vi "Read Motor Temperature.vi"(11 "Thermocouple in":refnum<class "Thermocouple.lvclass">) -> (2 "Motor Temperature":dbl[unit]=273.15 min=-614.85 max=1161.15 format="%.6f", 3 "Thermocouple out":refnum<class "Thermocouple.lvclass">)   [LabVIEW 2013, in "Thermocouple.lvclass"]
uses:
  Thermocouple.lvclass
  Thermocouple.lvclass/Thermocouple.ctl
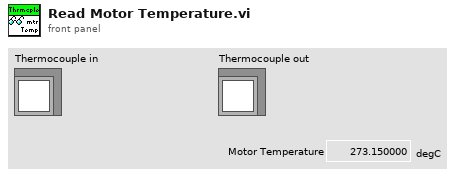
[diagram p1: front panel]
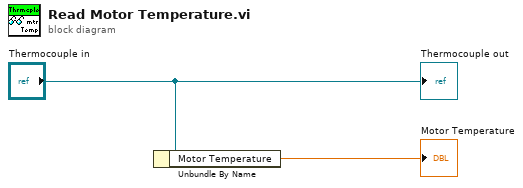
[diagram p0: block diagram]
diagram:
  n1 = Unbundle By Name("Thermocouple in") -> ("Motor Temperature"=→"Motor Temperature":dbl[unit])
  "Thermocouple out" <- "Thermocouple in"
